vi "Read Input Registers Request.vi"(8 "error in (no error)":errorcluster, 9 "number of registers":u16, 10 "starting address":u16) -> (0 "error out":errorcluster, 2 "Modbus data unit out":refnum<class "Modbus Data Unit (PDU).lvclass">)   [LabVIEW 2018, in "SubVIs.lvlib" / "Master Function Definition.lvlib"]
doc: "This VI forms a modbus data unit for reading multiple input registers"
uses:
  Master Function Definition.lvlib
  Modbus Data Unit (PDU).lvclass
  Modbus Data Unit (PDU).lvclass/Modbus Data Unit (PDU).ctl
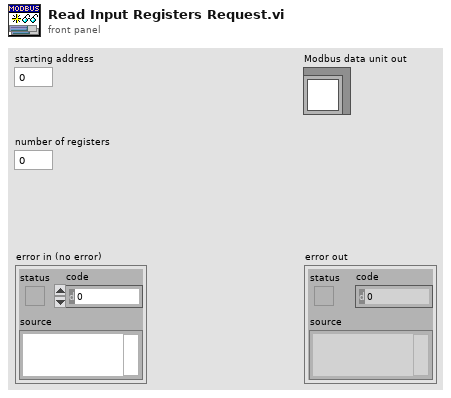
[diagram p1: front panel]
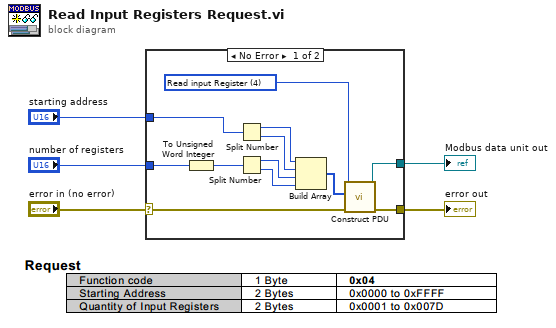
[diagram p0: block diagram]
diagram:
  n1 = case shown="No Error" "error in (no error)" {
    selector: "error in (no error)" -> [w6 w18]
    tunnel: [w17 w18] -> w5
    tunnel: "starting address" -> [w16 _]
    tunnel: [w15 _] -> w3
    tunnel: "number of registers" -> [w7 _]
    frame No Error {
      w9 = u8 4 items=["Read Discrete Inputs"=2, "Read Coils"=1, "Write Single Coil"=5, "Write Multiple Coils"=15, "Read input Register"=4, "Read Holding Registers"=3, "Write Single Register"=6, "Write Multiple Registers"=16, "Read/Write Multiple Registers"=23, "Mask Write Register"=22, "Read FIFO Queue"=24, "Read File Record"=20, "Write File Record"=21, "Read Exception Status"=7, "Diagnostic"=8, "Get Com Event Counter"=11, "Get Com Event Log"=12, "Report Slave ID"=17, "Read Device Identification"=43] ("Function")
      n2 = To Unsigned Word Integer(number=w7) -> (unsigned 16bit integer=w8:u16)
      n3 = Split Number(x=w16) -> (hi(x)=w11:u8, lo(x)=w12:u8)
      n4 = Split Number(x=w8) -> (hi(x)=w13:u8, lo(x)=w14:u8)
      n5 = Build Array(w11, w12, w13, w14) -> (w10:u8[])
      n6 = call "Construct PDU.vi"("error in (no error)"=w6, "data"=w10, "function"=w9) -> ("error out"=w17:errorcluster, "Modbus data unit out"=w15:refnum<class "Modbus Data Unit (PDU).lvclass">)  [unwired: 7 in]
    }
    frame Error {
    }
  }
  "error out" <- w5
  "Modbus data unit out" <- w3
